vi "ClsSendCmds_Array.vi"(8 "error in (no error)":errorcluster, 10 "InitCommandArray":string[](array[string]), 11 "Connection Out in":u32) -> (0 "error out":errorcluster, 2 "Array of Command Responses":string[](array[string]), 3 "Connection Out out":u32)   [LabVIEW 2015]
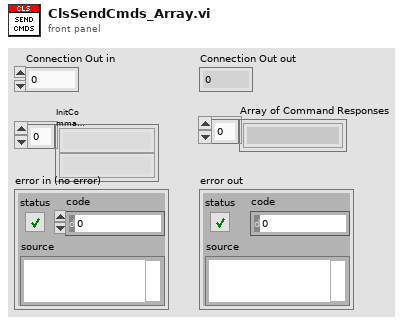
[diagram p1: front panel]
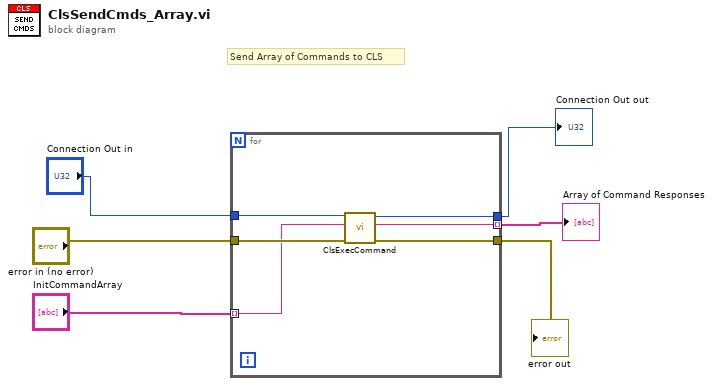
[diagram p0: block diagram]
diagram:
  # "Send Array of Commands to CLS"
  n1 = for {
    tunnel: "error in (no error)" -> [w12]
    tunnel: [w11] -> w3
    tunnel: [w10] -> w4
    tunnel: "Connection Out in" -> [w9]
    tunnel: "InitCommandArray" -> [w7] mode=indexing
    tunnel: [w8] -> w1 mode=indexing
    n2 = call "ClsExecCommand.vi"("error in (no error)"=w12, "Command In"=w7, "Connection In"=w9) -> ("error out"=w11:errorcluster, "Command Response"=w8:string, "Connection Out"=w10:u32)  [unwired: 6 in]
  }
  "Connection Out out" <- w4
  "error out" <- w3
  "Array of Command Responses" <- w1
